vi "healthcheckExample_S.vi"(1 "weight":string, 2 "rfid":string) -> (0 "Boolean":bool=TRUE)   [LabVIEW 2019]
doc: "The threshold to determine whether the bird is unhealthy or not (currently determined by weight, and whether the weight exceeds a certain threshold)\n\nIf threshold is exceeded, telegram message should be sent"
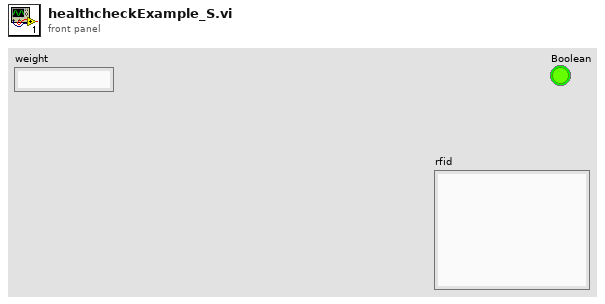
[diagram p1: front panel]
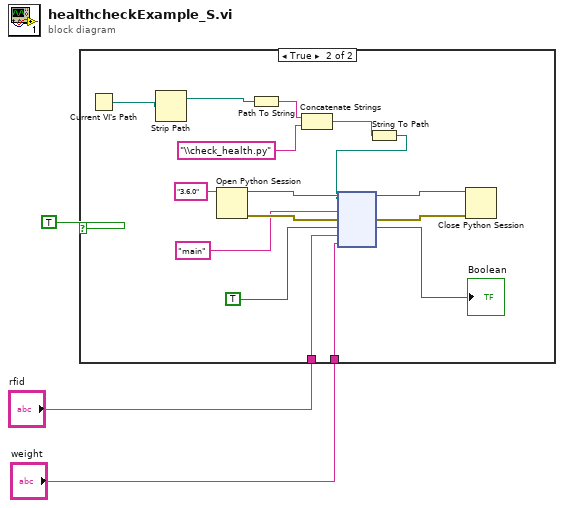
[diagram p0: block diagram]
diagram:
  n1 = case shown="True" TRUE {
    tunnel: "rfid" -> [_ w13]
    tunnel: "weight" -> [_ w4]
    frame False {
    }
    frame True {
      n2 = Current VI's Path() -> (path=w12:path)
      n3 = Strip Path(path=w12) -> (stripped path=w11:path)  [unwired: 1 out]
      n4 = Open Python Session(python version="3.6.0" ("Python version")) -> (session out=w19:refnum<k35>, error out=w18:errorcluster)  [unwired: 2 in]
      n5 = Path To String(path=w11) -> (string=w9:string)
      n6 = Concatenate Strings(w9, "\\check_health.py") -> (w8:string)
      n7 = String To Path(string=w8) -> (path=w7:path)
      n8 = node(w19, w7, "main" ("function name"), w18, TRUE, w13, w4) -> (w16:refnum<k35>, w17:errorcluster, →"Boolean":bool)  [unwired: 2 in, 2 out]
      n9 = Close Python Session(session in=w16, error in=w17) -> ()  [unwired: 1 out]
    }
  }
